vi "Menu_LV Class Control.vi"(11 "Affected Items Out":T1) -> (3 "Menu Items To Add":T2(array[cluster]))   [LabVIEW 2023]
uses:
  top/BundleMagic.ctl
panel:
  out "Enabled Status":enum8{"Enabled", "Disabled"}[](array[ring])
  out "Menu Item Display Name":string[](array[string])
  out "Position In Menu":T3(array[cluster])
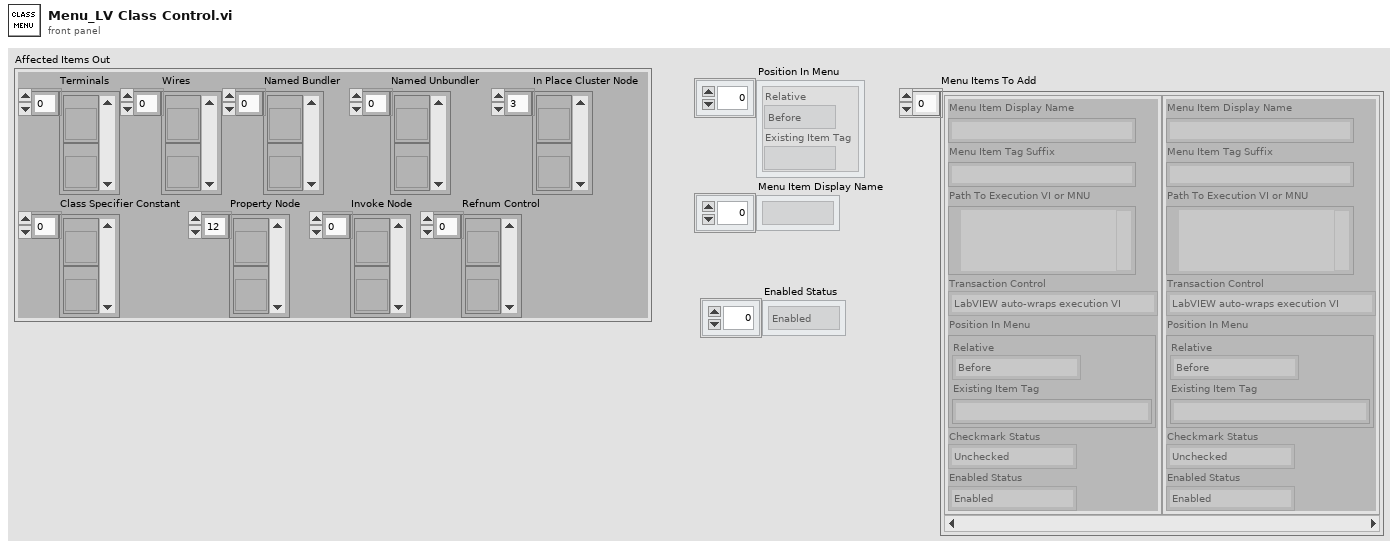
[diagram p1: front panel]
types:
  T1 = typedef "BundleMagic.ctl" = cluster{"Terminals":refnum<vi>[], "Wires":refnum<vi>[], "Named Bundler":refnum<vi>[], "Named Unbundler":refnum<vi>[], "In Place Cluster Node":refnum<vi>[], "Class Specifier Constant":refnum<vi>[], "Property Node":refnum<vi>[], "Invoke Node":refnum<vi>[], "Refnum Control":refnum<vi>[]}
  T2 = cluster{"Menu Item Display Name":string, "Menu Item Tag Suffix":string, "Path To Execution VI or MNU":path, "Transaction Control":enum8{"LabVIEW auto-wraps execution VI", "Execution VI will define if needed"}, "Position In Menu":cluster{"Relative":enum8{"Before", "Instead of", "After", "Into Submenu"}, "Existing Item Tag":string}, "Checkmark Status":enum8{"Unchecked", "Checked"}, "Enabled Status":enum8{"Enabled", "Disabled"}}[]
  T3 = cluster{"Relative":enum8{"Before", "Instead of", "After", "Into Submenu"}, "Existing Item Tag":string}[]
  T4 = enum16{"[NONE]", "Wire Bundle", "Wire Unbundle", "Terminal Unbundle", "Terminal Bundle", "Bundler Insert", "Bundler Remove", "Bundler Remove Unwired", "Bundler Rearrange", "In Place Insert", "In Place Remove", "In Place Remove Unwired", "In Place Rearrange", "Wire Properties", "Wire Method", "Terminal Properties", "Terminal Method", "Properties Insert", "Properties Remove", "Properties Remove Unwired", "Properties Rearrange", "Method Change", "Class for Constant", "Class For Control", "Class For Node", "Class Name to Clipboard"}[]
  T5 = cluster{"Menu Item Display Name":string, "Menu Item Tag Suffix":string, "Path To Execution VI or MNU":path, "Transaction Control":enum8{"LabVIEW auto-wraps execution VI", "Execution VI will define if needed"}, "Position In Menu":cluster{"Relative":enum8{"Before", "Instead of", "After", "Into Submenu"}, "Existing Item Tag":string}, "Checkmark Status":enum8{"Unchecked", "Checked"}, "Enabled Status":enum8{"Enabled", "Disabled"}}
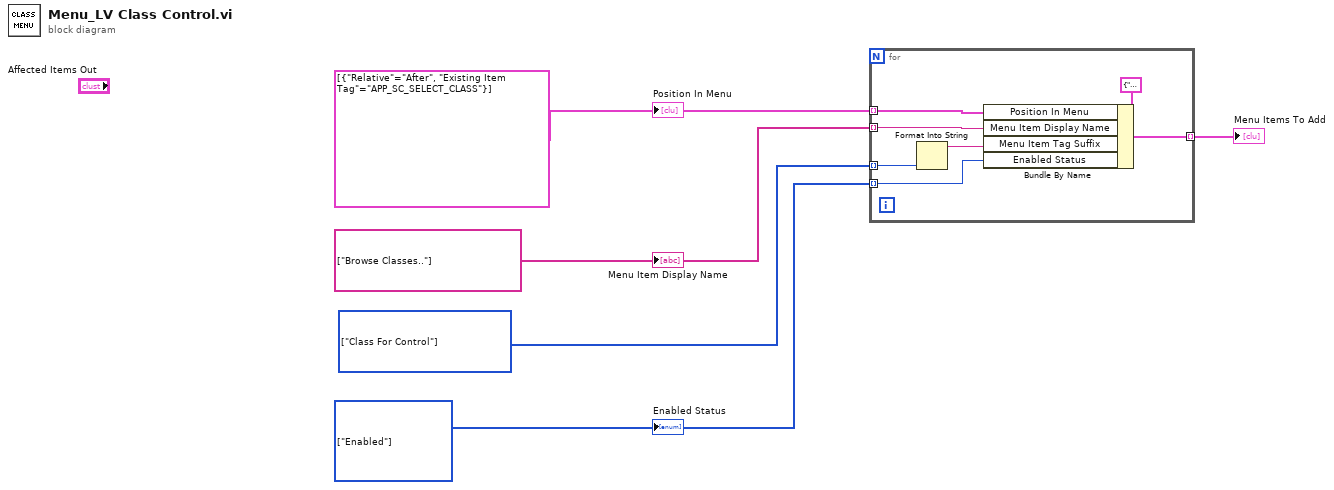
[diagram p0: block diagram]
diagram:
  w2 = enum8{"Enabled", "Disabled"}[] [enum."Enabled"] items=["Enabled", "Disabled"]
  w5 = T3 [{"Relative"=enum."After", "Existing Item Tag"="APP_SC_SELECT_CLASS"}]
  w3 = T4 [enum."Class For Control"] items=["[NONE]", "Wire Bundle", "Wire Unbundle", "Terminal Unbundle", "Terminal Bundle", "Bundler Insert", "Bundler Remove", "Bundler Remove Unwired", "Bundler Rearrange", "In Place Insert", "In Place Remove", "In Place Remove Unwired", "In Place Rearrange", "Wire Properties", "Wire Method", "Terminal Properties", "Terminal Method", "Properties Insert", "Properties Remove", "Properties Remove Unwired", "Properties Rearrange", "Method Change", "Class for Constant", "Class For Control", "Class For Node", "Class Name to Clipboard"]
  w4 = string[] ["Browse Classes.."]
  n1 = for {
    tunnel: [w12] -> w1 mode=indexing
    tunnel: w4 -> [w11] mode=indexing
    tunnel: w3 -> [w6] mode=indexing
    tunnel: w5 -> [w9] mode=indexing
    tunnel: w2 -> [w8] mode=indexing
    n2 = Format Into String(w6) -> (resulting string=w7:string)  [unwired: 3 in, 1 out]
    n3 = Bundle By Name(cluster=T5 {"Menu Item Display Name"="", "Menu Item Tag Suffix"="", "Path To Execution VI or MNU"=path "", "Transaction Control"=enum."LabVIEW auto-wraps execution VI", "Position In Menu"={"Relative"=enum."Before", "Existing Item Tag"=""}, "Checkmark Status"=enum."Unchecked", "Enabled Status"=enum."Enabled"} ("Cluster"), "Position In Menu"=w9, "Menu Item Display Name"=w11, "Menu Item Tag Suffix"=w7, "Enabled Status"=w8) -> (w12:T5)
  }
  "Menu Items To Add" <- w1
  "Position In Menu" <- w5
  "Menu Item Display Name" <- w4
  "Enabled Status" <- w2
